vi "Config Current.vi"(0 "VISA resource name":refnum<visa-resource-name>, 1 "Element (0: ALL)":u16(ring) items=["All", "Element 1", "Element 2", "Element 3", "Element 4"], 5 "A Terminal (0: 5A)":u16(ring) items=["5A", "20A", "Sensor"], 7 "A Range (7:10)":u16(ring)=7 items=["AUTO", "0.1", "0.2", "0.4", "1", "2", "4", "10", "20", "40", "100"], 11 "error in (no error)":errorcluster, 12 "A Sensor Ratio(mV/A) (10)":dbl=10.0 min=0.0001 max=99999.9999 step=0.0001 format="%.4f") -> (4 "VISA resource name out":refnum<visa-resource-name>, 15 "error out":errorcluster)   [LabVIEW 2014, in "Yokogawa.lvlib" / "Yokogawa PZ4000.lvlib"]
doc: "This VI sends the Current Configure command to the PZ4000 series.\nConfigure Control Functions are Selects the Current Terminal, Current Range and Sensor Ratio."
uses:
  Yokogawa PZ4000.lvlib
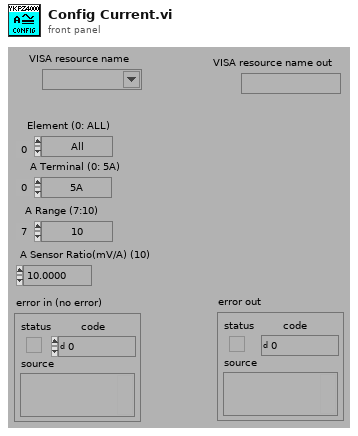
[diagram p1: front panel]
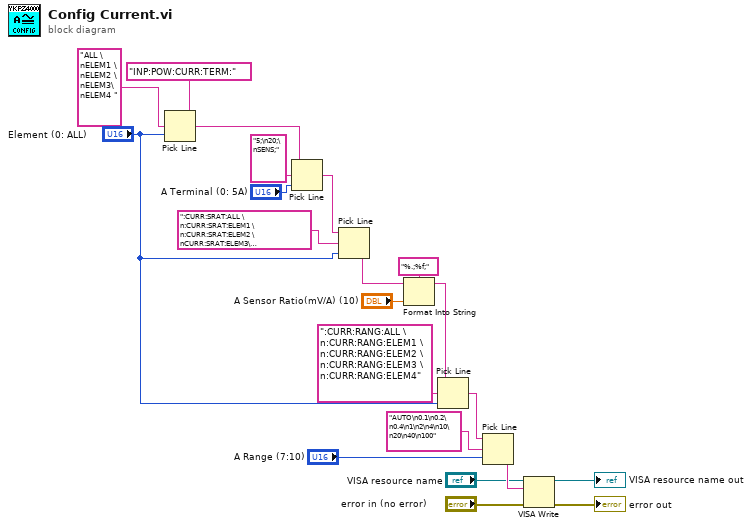
[diagram p0: block diagram]
diagram:
  n1 = Pick Line(string ("")="INP:POW:CURR:TERM:", multi-line string="ALL \nELEM1 \nELEM2 \nELEM3\nELEM4 ", line index="Element (0: ALL)") -> (output string=w12:string)
  n2 = Pick Line(string ("")=w12, multi-line string="5;\n20;\nSENS;", line index="A Terminal (0: 5A)") -> (output string=w11:string)
  n3 = Pick Line(string ("")=w11, multi-line string=":CURR:SRAT:ALL \n:CURR:SRAT:ELEM1 \n:CURR:SRAT:ELEM2 \nCURR:SRAT:ELEM3\nCURR:SRAT:ELEM4 ", line index="Element (0: ALL)") -> (output string=w8:string)
  n4 = Format Into String(format string="%.;%f;", initial string=w8, "A Sensor Ratio(mV/A) (10)") -> (resulting string=w4:string)  [unwired: 1 in, 1 out]
  n5 = Pick Line(string ("")=w4, multi-line string=":CURR:RANG:ALL \n:CURR:RANG:ELEM1 \n:CURR:RANG:ELEM2 \n:CURR:RANG:ELEM3 \n:CURR:RANG:ELEM4", line index="Element (0: ALL)") -> (output string=w20:string)
  n6 = Pick Line(string ("")=w20, multi-line string="AUTO\n0.1\n0.2\n0.4\n1\n2\n4\n10\n20\n40\n100", line index="A Range (7:10)") -> (output string=w16:string)
  n7 = VISA Write(VISA resource name="VISA resource name", write buffer=w16, error in (no error)="error in (no error)") -> (VISA resource name out=→"VISA resource name out":refnum<visa-resource-name>, error out=→"error out":errorcluster)  [unwired: 1 out]
